vi "Menu_Refnum Terminal.vi"(11 "Affected Items":T1) -> (3 "Menu Items To Add":T2(array[cluster]))   [LabVIEW 2023]
uses:
  top/BundleMagic.ctl
  controls/action enum.ctl
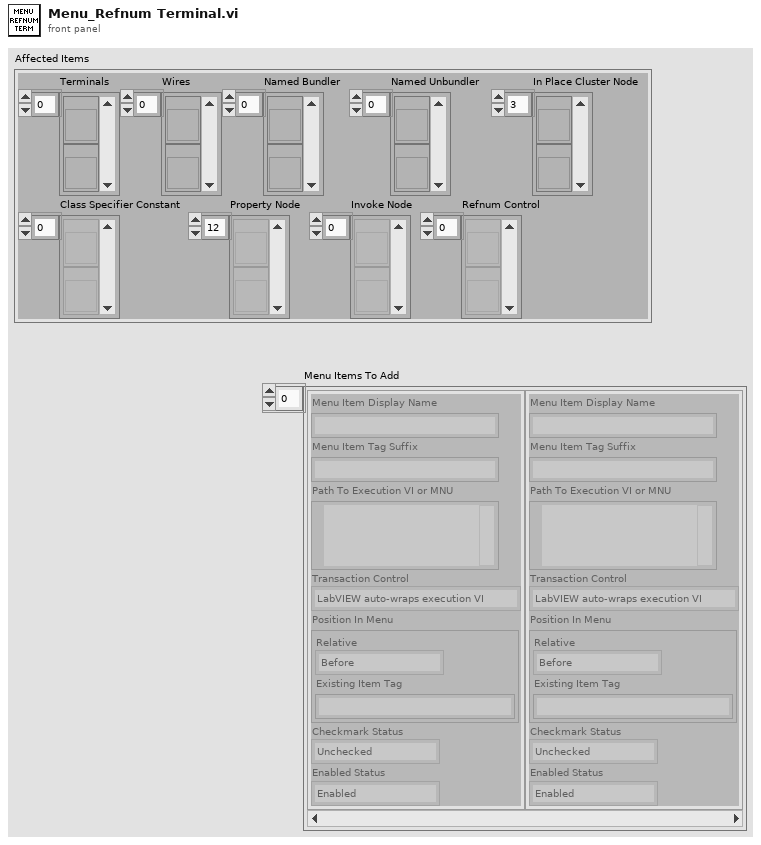
[diagram p1: front panel]
types:
  T1 = typedef "BundleMagic.ctl" = cluster{"Terminals":refnum<vi>[], "Wires":refnum<vi>[], "Named Bundler":refnum<vi>[], "Named Unbundler":refnum<vi>[], "In Place Cluster Node":refnum<vi>[], "Class Specifier Constant":refnum<vi>[], "Property Node":refnum<vi>[], "Invoke Node":refnum<vi>[], "Refnum Control":refnum<vi>[]}
  T2 = cluster{"Menu Item Display Name":string, "Menu Item Tag Suffix":string, "Path To Execution VI or MNU":path, "Transaction Control":enum8{"LabVIEW auto-wraps execution VI", "Execution VI will define if needed"}, "Position In Menu":cluster{"Relative":enum8{"Before", "Instead of", "After", "Into Submenu"}, "Existing Item Tag":string}, "Checkmark Status":enum8{"Unchecked", "Checked"}, "Enabled Status":enum8{"Enabled", "Disabled"}}[]
  T3 = typedef "action enum.ctl" = enum16{"[NONE]", "APP_SEPARATOR", "Wire Bundle", "Wire Unbundle", "Terminal Unbundle", "Terminal Bundle", "Bundler Move Up", "Bundler Move Down", "Bundler Insert", "Bundler Remove", "Bundler Remove Unwired", "Bundler Rearrange", "In Place Insert", "In Place Remove", "In Place Remove Unwired", "In Place Rearrange", "Wire Properties", "Wire Method", "Terminal Properties", "Terminal Method", "Property Move Up", "Property Move Down", "Properties Insert", "Properties Remove", "Properties Remove Unwired", "Properties Rearrange", "Method Change", "Class For Constant", "Class For Control", "Class For Node", "Class Name to Clipboard"}
  T4 = cluster{"Relative":enum8{"Before", "Instead of", "After", "Into Submenu"}, "Existing Item Tag":string}
  T5 = cluster{"Relative":enum8{"Before", "Instead of", "After", "Into Submenu"}, "Existing Item Tag":string}[]
  T6 = cluster{"Menu Item Display Name":string, "Menu Item Tag Suffix":string, "Path To Execution VI or MNU":path, "Transaction Control":enum8{"LabVIEW auto-wraps execution VI", "Execution VI will define if needed"}, "Position In Menu":cluster{"Relative":enum8{"Before", "Instead of", "After", "Into Submenu"}, "Existing Item Tag":string}, "Checkmark Status":enum8{"Unchecked", "Checked"}, "Enabled Status":enum8{"Enabled", "Disabled"}}
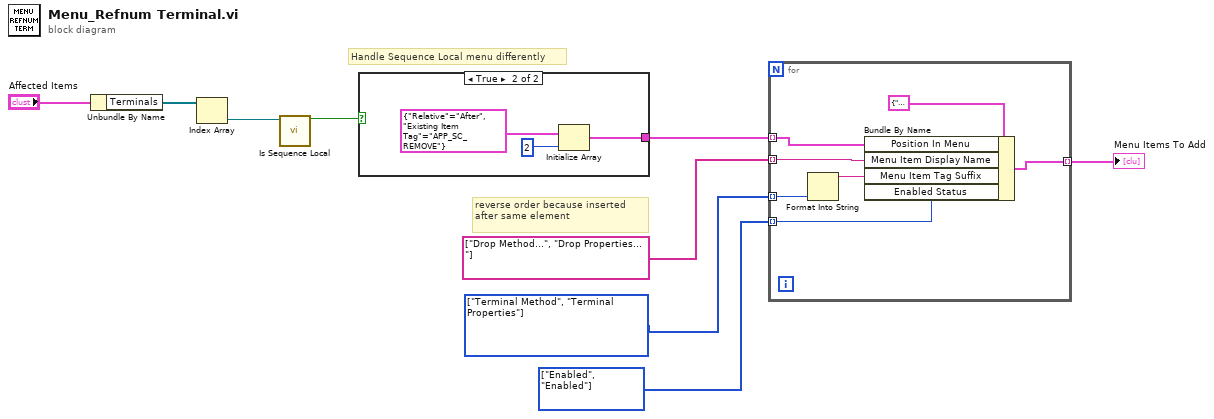
[diagram p0: block diagram]
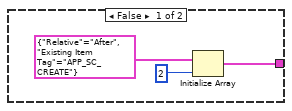
[diagram p2: hidden frame]
diagram:
  w1 = T3[] [enum."Terminal Method", enum."Terminal Properties"] items=["[NONE]", "APP_SEPARATOR", "Wire Bundle", "Wire Unbundle", "Terminal Unbundle", "Terminal Bundle", "Bundler Move Up", "Bundler Move Down", "Bundler Insert", "Bundler Remove", "Bundler Remove Unwired", "Bundler Rearrange", "In Place Insert", "In Place Remove", "In Place Remove Unwired", "In Place Rearrange", "Wire Properties", "Wire Method", "Terminal Properties", "Terminal Method", "Property Move Up", "Property Move Down", "Properties Insert", "Properties Remove", "Properties Remove Unwired", "Properties Rearrange", "Method Change", "Class For Constant", "Class For Control", "Class For Node", "Class Name to Clipboard"] ("Array")
  w2 = enum8{"Enabled", "Disabled"}[] [enum."Enabled", enum."Enabled"] items=["Enabled", "Disabled"] ("Enabled Status")
  # "reverse order because inserted after same element"
  # "Handle Sequence Local menu differently"
  n1 = Unbundle By Name("Affected Items") -> ("Terminals"=w6:refnum<vi>[])
  n2 = Index Array(array=w6) -> (element=w3:refnum<vi>)  [unwired: 1 in]
  n3 = call "Is Sequence Local.vi"("Terminal in"=w3) -> ("Is Seq Local?"=w4:bool)  [unwired: 9 in, 1 out]
  n4 = case shown="True" w4 {
    tunnel: [w10 w13] -> w5
    frame False {
      n5 = Initialize Array(T4 {"Relative"=enum."After", "Existing Item Tag"="APP_SC_CREATE"} ("Position In Menu"), 2) -> (w10:T5)
    }
    frame True {
      n6 = Initialize Array(T4 {"Relative"=enum."After", "Existing Item Tag"="APP_SC_REMOVE"} ("Position In Menu"), 2) -> (w13:T5)
    }
  }
  n7 = for {
    tunnel: [w20] -> w9 mode=indexing
    tunnel: w5 -> [w18] mode=indexing
    tunnel: string[] ["Drop Method...", "Drop Properties..."] -> [w21] mode=indexing
    tunnel: w2 -> [w19] mode=indexing
    tunnel: w1 -> [w17] mode=indexing
    n8 = Format Into String(w17) -> (resulting string=w16:string)  [unwired: 3 in, 1 out]
    n9 = Bundle By Name(cluster=T6 {"Menu Item Display Name"="", "Menu Item Tag Suffix"="", "Path To Execution VI or MNU"=path "", "Transaction Control"=enum."LabVIEW auto-wraps execution VI", "Position In Menu"={"Relative"=enum."Before", "Existing Item Tag"=""}, "Checkmark Status"=enum."Unchecked", "Enabled Status"=enum."Enabled"} ("Cluster"), "Position In Menu"=w18, "Menu Item Display Name"=w21, "Menu Item Tag Suffix"=w16, "Enabled Status"=w19) -> (w20:T6)
  }
  "Menu Items To Add" <- w9
